vi "DistToObstNearwAng2.vi"(2 "Boat Point":T1 {"North" format="%#_10f"; "East" format="%#_8f"}, 3 "Segment Point 2":T1 {"North" format="%#_10f"; "East" format="%#_8f"}, 4 "Segment Point 1":T1 {"North" format="%#_10f"; "East" format="%#_8f"}) -> (0 "Distance between boat and segment":dbl, 1 "Angle to Obstacle, Trig Abs":dbl(knob))   [LabVIEW 2013]
doc: "Takes in a segment, and a boat point, and returns the distance between the segment and the boat, and the angle to the segment or the nearest point. For obstacle avoidance. There may be a failure case where division of absolute angles fails when done across zero, it has not yet been found."
uses:
  Data/TypeDefs/UTM Location.ctl
  Utilities/Math/Angles/Angle/Angle.lvclass
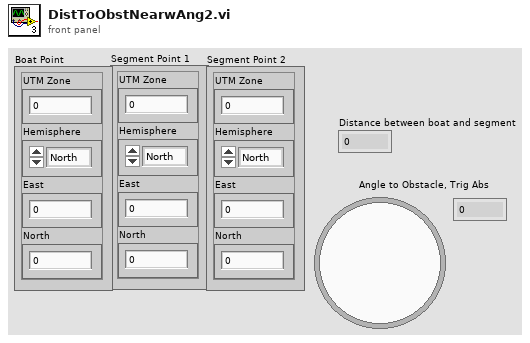
[diagram p1: front panel]
types:
  T1 = typedef "UTM Location.ctl" = cluster{"UTM Zone":dbl, "Hemisphere":enum16{"North", "South"}, "East":dbl, "North":dbl}
diagram:
  # "Law of cosines would have been better to use in retrospect"
  # "There may be a failure case where the subtraction of absolute angles fails when done across zero, haven't been able to find it"
  # "Why the distance works, acute case:\nthe difference of the abs angles is the the angle from the segment to the boat from point 2\nthe hyp of that interior triangle is the distance between them\nsin(x) times that hyp is the opp length from the boat to the segment\nObtuse case: gets distance to obtuse angle vertex\n\nWhy the angle works for the acute case:\nCalcs the line perpendicular to the segment line, adds or subtracts pi/2 based on the relative\nabs angles of the segment and the boat.\n\nAngle for obtuse case: abs angle from obtuse angle vertex \n\nNote: Obtuse triangle only relevant when a segment point is an obtuse vertex."
  # "Checks for right or obtuse segment point"
  n1 = call "Initialize.vi"() -> ()  [unwired: 10 in, 2 out]
  n2 = call "CalcTrigAbsAngle.vi"("Point 2"="Boat Point", "Point 1"="Segment Point 1") -> ("Angle between points (rad)"=w8:dbl)  [unwired: 9 in]
  n3 = call "DistBetweenPoints.vi"("UTM Location 2"="Boat Point", "UTM Location"="Segment Point 1") -> ("Numeric"=w15:dbl)
  n4 = call "CalcTrigAbsAngle.vi"("Point 2"="Segment Point 2", "Point 1"="Segment Point 1") -> ("Angle between points (rad)"=w9:dbl)  [unwired: 9 in]
  n5 = call "CalcTrigAbsAngle.vi"("Point 2"="Segment Point 1", "Point 1"="Segment Point 2") -> ("Angle between points (rad)"=w7:dbl)  [unwired: 9 in]
  n6 = call "CalcTrigAbsAngle.vi"("Point 2"="Boat Point", "Point 1"="Segment Point 2") -> ("Angle between points (rad)"=w6:dbl)  [unwired: 9 in]
  n7 = call "DistBetweenPoints.vi"("UTM Location 2"="Boat Point", "UTM Location"="Segment Point 2") -> ("Numeric"=w18:dbl)
  n8 = call "SimpleAngleDifference.vi"("Report in degrees? (False = Radians, default = True)"=FALSE, "Angle 2"=w8, "Angle 1"=w9) -> ("Absolute Difference"=w3:dbl)  [unwired: 7 in, 1 out]
  n9 = call "SimpleAngleDifference.vi"("Report in degrees? (False = Radians, default = True)"=FALSE, "Angle 2"=w6, "Angle 1"=w7) -> ("Absolute Difference"=w4:dbl, "Difference"=w5:dbl)  [unwired: 7 in]
  n10 = Greater Or Equal?(x=w3, y=1.5707963267948966) -> (x >= y?=w11:bool)
  n11 = Greater Or Equal?(x=w4, y=1.5707963267948966) -> (x >= y?=w10:bool)
  n12 = Or(x=w11, y=w10) -> (x .or. y?=w19:bool)
  n13 = case shown="False" w19 {
    tunnel: w4 -> [w34 _]
    tunnel: w18 -> [w33 w42]
    tunnel: [w32 w41] -> w17
    tunnel: [w24 w39] -> w16
    tunnel: w5 -> [w23 _]
    tunnel: w7 -> [w22 _]
    tunnel: w10 -> [_ w43]
    tunnel: w6 -> [_ w40]
    tunnel: w15 -> [_ w38]
    tunnel: w8 -> [_ w37]
    frame False {
      # "Gets the line perpendicular to the segment,\nand the chooses direction based on relative\nabs angles"
      n14 = Sine(x=w34) -> (sin(x)=w35:dbl)
      n15 = Multiply(x=w35, y=w33) -> (x*y=w36:dbl)
      n16 = Absolute Value(x=w36) -> (abs(x)=w32:dbl)
      n17 = Add(x=1.5707963267948966, y=w22) -> (x+y=w26:dbl)
      n18 = Subtract(x=w22, y=1.5707963267948966) -> (x-y=w28:dbl)
      n19 = Less Than 0?(x=w23) -> (x < 0?=w29:bool)
      n20 = Quotient & Remainder(x=w26, y=6.283185307179586) -> (x-y*floor(x/y)=w25:dbl)  [unwired: 1 out]
      n21 = Select(t=w25, s=w29, f=w28) -> (s? t:f=w24:dbl)
    }
    frame True {
      # "Both can't be obtuse.  If one is, takes\ndistance and abs ang from it as the returns"
      n22 = case shown="True" w43 {
        tunnel: w42 -> [_ w47]
        tunnel: [w45 w47] -> w41
        tunnel: w40 -> [_ w46]
        tunnel: [w44 w46] -> w39
        tunnel: w38 -> [w45 _]
        tunnel: w37 -> [w44 _]
        frame False {
        }
        frame True {
        }
      }
    }
  }
  "Distance between boat and segment" <- w17
  "Angle to Obstacle, Trig Abs" <- w16
